vi "subNextStatus.vi"(2 "Markov Matrix":dbl[][](array[numeric]), 3 "Status":i32) -> (0 "next probability(max)":dbl, 1 "next status(max)":i32)   [LabVIEW 2014]
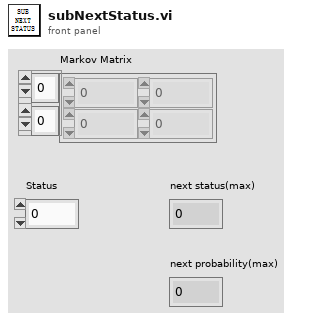
[diagram p1: front panel]
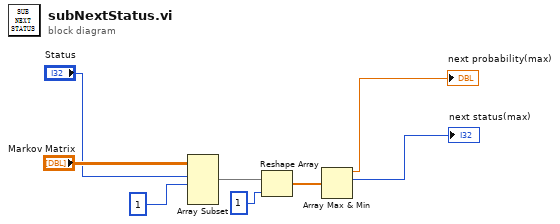
[diagram p0: block diagram]
diagram:
  n1 = Array Subset(array="Markov Matrix", index (row)="Status", length (row)=1 ("length")) -> (w6:dbl[][])  [unwired: 2 in]
  n2 = Reshape Array(w6, 1 ("dimension size")) -> (w3:dbl[])
  n3 = Array Max & Min(array=w3) -> (max value=→"next probability(max)":dbl, max index (indices)=→"next status(max)":i32)  [unwired: 2 out]
